vi "H(z)toH(w)-CascadeIIR.vi"(0 "IIR Filter Cluster":T1 {"Forward Coefficients" format="%0.4f"; "Reverse Coefficients" format="%0.4f"}, 1 "FFT size":i32=1024) -> (2 "Mag H(w)":dbl[](array[numeric]) format="%0.2f", 3 "Phase H(w)":dbl[](array[numeric]) format="%0.2f", 4 "df":dbl format="%0.2f")   [LabVIEW 2020]
uses:
  <vilib>/Analysis/2dsp.llb/Real FFT.vi
  <vilib>/Analysis/NI_AALPro.lvlib
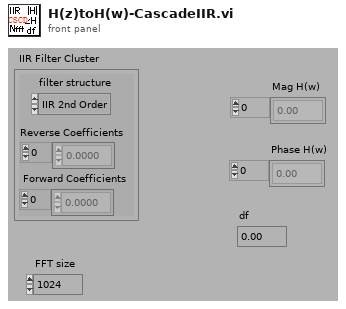
[diagram p1: front panel]
types:
  T1 = cluster{"filter structure":enum32{"IIR 2nd Order", "IIR 4th Order"}, "Reverse Coefficients":dbl[], "Forward Coefficients":dbl[]}
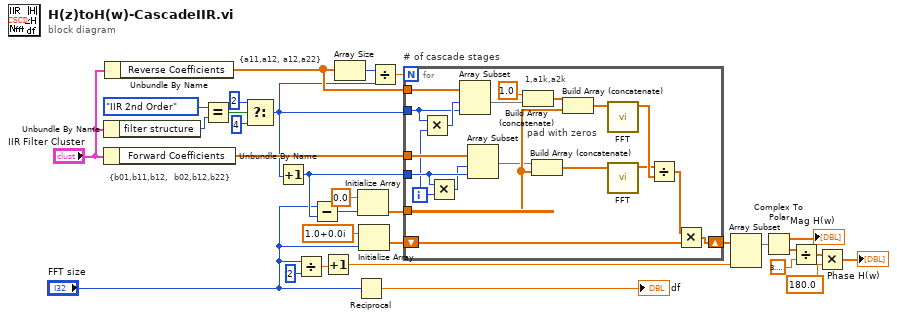
[diagram p0: block diagram]
diagram:
  # "{a11,a12, a12,a22}"
  # "{b01,b11,b12,  b02,b12,b22}"
  # "# of cascade stages"
  n1 = Unbundle By Name("IIR Filter Cluster") -> ("filter structure"=w5:enum32{"IIR 2nd Order", "IIR 4th Order"})
  n2 = Unbundle By Name("IIR Filter Cluster") -> ("Forward Coefficients"=w29:dbl[])
  n3 = Unbundle By Name("IIR Filter Cluster") -> ("Reverse Coefficients"=w26:dbl[])
  n4 = Equal?(x=enum32{"IIR 2nd Order", "IIR 4th Order"}."IIR 2nd Order" ("filter structure"), y=w5) -> (x = y?=w2:bool)
  n5 = Select(t=2, s=w2, f=4) -> (s? t:f=w1:i32)
  n6 = Increment(x=w1) -> (x+1=w13:i32)
  n7 = Divide(x="FFT size", y=2) -> (x/y=w22:dbl)
  n8 = Subtract(x="FFT size", y=w13) -> (x-y=w15:i32)
  n9 = Increment(x=w22) -> (x+1=w21:dbl)
  n10 = Array Size(array=w26) -> (size(s)=w30:i32)
  n11 = Reciprocal(x="FFT size") -> (1/x=→"df":dbl)
  n12 = Initialize Array(0.0, w15) -> (w14:dbl[])
  n13 = Initialize Array(cdb 1.0+0.0i, "FFT size") -> (w24:cdb[])
  n14 = Divide(x=w30, y=w1) -> (x/y=w27:dbl)
  n15 = for {
    N: w27 -> [_]
    shift-right: [w40] -> w19
    shift-left: w24 -> [w38]
    tunnel: w1 -> [w46]
    tunnel: w26 -> [w45]
    tunnel: w29 -> [w44]
    tunnel: w13 -> [w43]
    tunnel: w14 -> [w37]
    i -> [w41]
    # "pad with zeros"
    # "1,a1k,a2k"
    n16 = Multiply(x=w46, y=w41) -> (x*y=w47:i32)
    n17 = Multiply(x=w43, y=w41) -> (x*y=w42:i32)
    n18 = Array Subset(array=w45, index=w47, length=w46) -> (w49:dbl[])
    n19 = Array Subset(array=w44, index=w42, length=w43) -> (w34:dbl[])
    n20 = Build Array (concatenate)(1.0, w49) -> (w35:dbl[])
    n21 = Build Array (concatenate)(w34, w37) -> (w33:dbl[])
    n22 = Build Array (concatenate)(w35, w37) -> (w36:dbl[])
    n23 = call-poly <vilib>:"FFT.vi"("X"=w36) -> ("FFT {X}"=w32:cdb[])  [unwired: 9 in, 1 out]
    n24 = call-poly <vilib>:"FFT.vi"("X"=w33) -> ("FFT {X}"=w31:cdb[])  [unwired: 9 in, 1 out]
    n25 = Divide(x=w31, y=w32) -> (x/y=w39:cdb[])
    n26 = Multiply(x=w39, y=w38) -> (x*y=w40:cdb[])
  }
  n27 = Array Subset(array=w19, length=w21) -> (w18:cdb[])  [unwired: 1 in]
  n28 = Complex To Polar(r * e^(i*theta)=w18) -> (r=→"Mag H(w)":dbl[], theta=w8:dbl[])
  n29 = Divide(x=w8, y=3.141592653589793) -> (x/y=w9:dbl[])
  n30 = Multiply(x=w9, y=180.0) -> (x*y=→"Phase H(w)":dbl[])
